vi "wd_clearBuffer.vi"(8 "error in (no error)":errorcluster, 11 "Excel refnum in":T1) -> (0 "error out":errorcluster, 3 "Excel refnum out":T1)   [LabVIEW 2017, in "NI_ExcelFile.lvlib"]
uses:
  <vilib>/express/express shared/NI_ExcelFile/NI_ExcelFile.lvlib
  <vilib>/express/express shared/NI_ExcelFile/Ctrls/ExcelRefnum.ctl
  <vilib>/express/express shared/NI_ExcelFile/Ctrls/MainData.ctl
  <vilib>/express/express shared/NI_ExcelFile/Ctrls/StreamMode.ctl
  <vilib>/express/express shared/NI_ExcelFile/Ctrls/TimeColumnMode.ctl
  <vilib>/express/express shared/NI_ExcelFile/Ctrls/FileAttribute.ctl
  <vilib>/express/express shared/NI_ExcelFile/Ctrls/Columns.ctl
  <vilib>/express/express shared/NI_ExcelFile/Ctrls/ColumnInfo.ctl
  <vilib>/express/express shared/NI_ExcelFile/Ctrls/DataType.ctl
  <vilib>/express/express shared/NI_ExcelFile/Ctrls/wd_recordInfo.ctl
  <vilib>/express/express shared/NI_ExcelFile/Ctrls/disk_TemplateFile.ctl
  <vilib>/express/express shared/NI_ExcelFile/Ctrls/meta_file.ctl
  <vilib>/express/express shared/NI_ExcelFile/Ctrls/meta_Block.ctl
  <vilib>/express/express shared/NI_ExcelFile/Ctrls/meta_BlockType.ctl
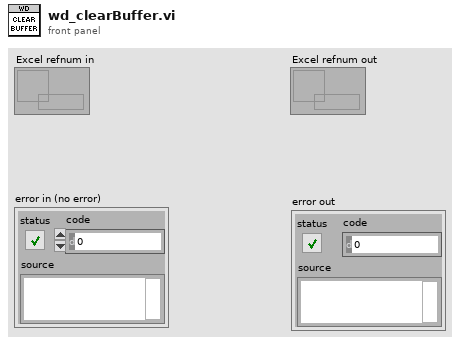
[diagram p1: front panel]
types:
  T1 = typedef "NI_ExcelFile.lvlib/ExcelRefnum.ctl" = refnum<data-value>
  T2 = typedef "NI_ExcelFile.lvlib/wd_recordInfo.ctl" = cluster{"ChannelIndex":u32, "StartIndex":u64, "Length":u64, "Previous":i32, "Next":i32}
  T3 = typedef "NI_ExcelFile.lvlib/Columns.ctl" = T4[]
  T4 = typedef "NI_ExcelFile.lvlib/ColumnInfo.ctl" = cluster{"Header":string, "Format":string, "DataType":T5, "Length":u64}
  T5 = typedef "NI_ExcelFile.lvlib/DataType.ctl" = enum16{"DDT", "WFM", "Array of STR", "Array of DBL", "Array of I8", "Array of I16", "Array of I32", "Array of I64", "Array of SGL", "Array of U8", "Array of U16", "Array of U32", "Array of U64", "Array of Time"}
  T6 = enum16{"open", "replace", "create", "open or create", "replace or create", "replace or create with confirmation"}
  T7 = typedef "NI_ExcelFile.lvlib/MainData.ctl" = cluster{"TargetFile":path, "StreamMode":T8, "Append?":bool, "ChunkSize":u64, "TimeColumnMode":T9, "TimestampFormat":string, "AbsoluteTime?":bool, "FileAttribute ":T10, "Column":T3, "FileRef":refnum<k1>, "MemoryRef":refnum<data-value>[], "RecordInfo":T2[], " ChannelPreviousInfo":u32[], "ChannelFirstRecord":u32[], "PredefinedFormattedValueLength":i64, "DiskTemplate":T11}
  T8 = typedef "NI_ExcelFile.lvlib/StreamMode.ctl" = enum16{"File", "Memory"}
  T9 = typedef "NI_ExcelFile.lvlib/TimeColumnMode.ctl" = enum16{"Empty", "OnePerCh", "One"}
  T10 = typedef "NI_ExcelFile.lvlib/FileAttribute.ctl" = cluster{"Creator":string, "Title":string, "SheetName":string}
  T11 = typedef "NI_ExcelFile.lvlib/disk_TemplateFile.ctl" = cluster{"XMLRef":refnum<file>[], "ZipPath":path, "MetaFile":T12, "TempFolder":path}
  T12 = typedef "NI_ExcelFile.lvlib/meta_file.ctl" = cluster{"Ref":refnum<file>, "NextRow":i32, "NextPosition":i64, "Block":T13[]}
  T13 = typedef "NI_ExcelFile.lvlib/meta_Block.ctl" = cluster{"Version":u16, "Type":T14, "Length":i32, "Data":string}
  T14 = typedef "NI_ExcelFile.lvlib/meta_BlockType.ctl" = enum16{"NITag", "File", "Column"}
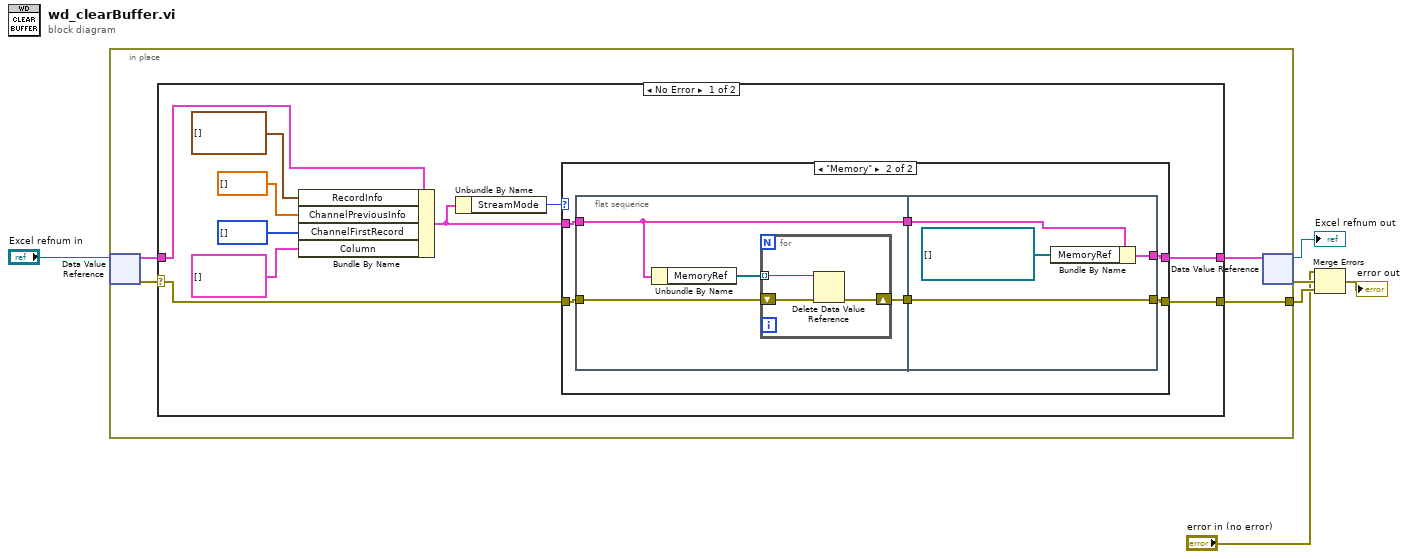
[diagram p0: block diagram]
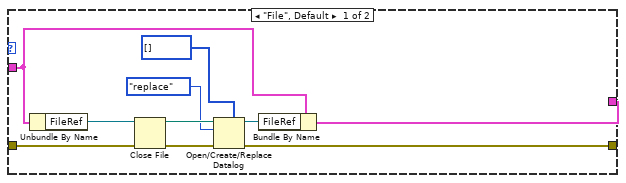
[diagram p2: hidden frame]
diagram:
  n1 = in-place {
    in-place-border: [w8] -> w3
    n2 = in-place-dvr #1("Excel refnum in") -> (w9:T7, w10:errorcluster)
    n3 = case shown="No Error" w10 {
      selector: w10 -> [w14 w48]
      tunnel: w9 -> [w15 w49]
      tunnel: [w13 w48] -> w8
      tunnel: [w12 w49] -> w7
      frame No Error {
        n4 = Bundle By Name(cluster=w15, "RecordInfo"=T2[] [], "ChannelPreviousInfo"=dbl[] [] ("Previous Info"), "ChannelFirstRecord"=i64[] [] ("Column first record"), "Column"=T3 [] ("Columns")) -> (w20:T7)
        n5 = Unbundle By Name(w20) -> ("StreamMode"=w19:T8)
        n6 = case shown="\"Memory\"" w19 {
          tunnel: w20 -> [w21 w36]
          tunnel: [w25 w35] -> w12
          tunnel: w14 -> [w24 w34]
          tunnel: [w22 w33] -> w13
          frame "File", Default {
            n7 = Unbundle By Name(w21) -> ("FileRef"=w30:refnum<k1>)
            n8 = Close File(refnum=w30, error in=w24) -> (path=w29:path, error out=w23:errorcluster)
            n9 = Open/Create/Replace Datalog(5:u8[] [] ("unsigned byte array"), 8:w23, 10:T6."replace" ("operation (0:open)"), 11:w29) -> (0:w22:errorcluster, 3:w27:refnum<k1>)  [unwired: 2 in, 1 out]
            n10 = Bundle By Name(cluster=w21, "FileRef"=w27) -> (w25:T7)
          }
          frame "Memory" {
            n11 = flat-sequence {
              tunnel: w36 -> [w37]
              tunnel: w34 -> [w39]
              tunnel: [w37] -> w32
              tunnel: [w38] -> w31
              tunnel: [w47] -> w33
              tunnel: [w44] -> w35
              tunnel: w32 -> [w45]
              tunnel: w31 -> [w47]
              frame #0 {
                n12 = Unbundle By Name(w37) -> ("MemoryRef"=w40:refnum<data-value>[])
                n13 = for {
                  tunnel: w40 -> [w43] mode=indexing
                  shift-right: [w41] -> w38
                  shift-left: w39 -> [w42]
                  n14 = Delete Data Value Reference(data value reference=w43, error in=w42) -> (error out=w41:errorcluster)  [unwired: 1 out]
                }
              }
              frame #1 {
                n15 = Bundle By Name(cluster=w45, "MemoryRef"=refnum<data-value>[] []) -> (w44:T7)
              }
            }
          }
        }
      }
      frame Error {
      }
    }
    n16 = in-place-dvr #1(w7) -> (→"Excel refnum out":T1, w2:errorcluster)
  }
  n17 = Merge Errors("error in (no error)", w2, w3) -> (→"error out":errorcluster)
